vi "Test CycloneDX BOM.vi"() -> ()   [LabVIEW 2017]
uses:
  CycloneDX/CycloneDX JSON/CycloneDX Types.ctl
  <vilib>/National Instruments/NIPM API (Beta)/_support/package attributes.ctl
  <vilib>/JKI/VIPM API/command-line/support/Library Contents Cluster_vipm_api.ctl
  CycloneDX/CycloneDX SBOM/CycloneDX SBOM.lvclass
  C:/LabVIEW Working Directory/labview-cyclonedx-sbom/Source/CycloneDX/CycloneDX JSON/CycloneDX JSON.lvclass
  CycloneDX/CycloneDX Component/CycloneDX Component.lvclass
  CycloneDX/CycloneDX JSON/CycloneDX JSON.lvclass
  <vilib>/JKI/VIPM API/VIPM API_vipm_api.lvlib
  <vilib>/National Instruments/NIPM API (Beta)/NIPM_API.lvlib
  VIP Support/VIP SBOM Support.lvlib
  NIPKG Support/NIPKG SBOM Support.lvlib
  <vilib>/JDP Science/JSONtext/JSONtext.lvlib
panel:
  out "error out":errorcluster
  out "JSON":string="{\r  \"bomFormat\":\"CycloneDX\",\r  \"specVersion\":\"1.5\",\r  \"serialNumber\":\"urn:uuid:dd314ffc-d076-4662-b32e-20b770deedce\",\r  \"metadata\":{\r    \"timestamp\":\"2024-08-06T15:38:24.581Z\",\r    \"manufacture\":{\"name\":\"MySoftwareCompany Ltd\"},\r    \"supplier\":{\"name\":\"MySoftwareCompany Ltd\"},\r    \"component\":{\r      \"type\":\"application\",\r      \"name\":\"softwarename\",\r      \"metadata\":{\r        \"component\":{\r          \"supplier\":{\"name\":\"MySoftwareCompany Ltd\"},\r          \"author\":{\"name\":\"MySoftwareCompany Ltd\"},\r          \"version\":\"1.0.0\",\r          \"description\":\"My Software Name - the best software available\",\r          \"cpe\":\"cpe:2.3:a:mysoftwarecompany:softwarename:1.2.219:*:*:*:*:*:*:*\"\r        }\r      }\r    }\r  },\r  \"components\":[\r    {\r      \"type\":\"library\",\r      \"name\":\"MGI Numeric\",\r      \"version\":\"1.1.0.2\",\r      \"publisher\":\"MGI\",\r      \"author\":\"MGI\",\r      \"purl\":\"pkg:vip/MGI/mgi_lib_numeric@1.1.0.2?repository_name=NI%20LabVIEW%20Tools%20Network\",\r      \"licenses\":[\r        {\r          \"id\":\"BSD-3-Clause\",\r          \"name\":\"BSD 3-Clause \\\"New\\\" or \\\"Revised\\\" License\"\r        }\r      ],\r      \"properties\":[\r        {\r          \"name\":\"packageName\",\r          \"value\":\"mgi_lib_numeric-1.1.0.2\"\r        },\r        {\r          \"name\":\"repositoryName\",\r          \"value\":\"NI LabVIEW Tools Network\"\r        }\r      ]\r    },\r    {\r      \"type\":\"platform\",\r      \"name\":\"ni-labview-2021-runtime-engine-x86\",\r      \"version\":\"21.1.0.49476-0+f324\",\r      \"author\":\"National Instruments\",\r      \"description\":\"The LabVIEW Runtime is a software add-on that enables engineers to run executables on a nondevelopment machine.\",\r      \"purl\":\"pkg:nipkg/National%20Instruments/ni-labview-2021-runtime-engine-x86@21.1.0.49476-0+f324\",\r      \"properties\":[\r        {\r          \"name\":\"maintainerEmail\",\r          \"value\":\"support@ni.com\"\r        },\r        {\r          \"name\":\"homepage\",\r          \"value\":\"https://www.ni.com\"\r        },\r        {\r          \"name\":\"displayVersion\",\r          \"value\":\"2021 SP1\"\r        },\r        {\r          \"name\":\"displayName\",\r          \"value\":\"LabVIEW Runtime (32-bit)\"\r        },\r        {\r          \"name\":\"architecture\",\r          \"value\":\"windows_x64\"\r        },\r        {\r          \"name\":\"packageSizeBytes\",\r          \"value\":\"29378434\"\r        },\r        {\r          \"name\":\"detailedDescription\",\r          \"value\":\"The LabVIEW Runtime enables you to run executables created with the LabVIEW Application Builder on machines that do not have LabVIEW installed. The LabVIEW Runtime includes the libraries and other files necessary to run basic application types built in LabVIEW.\"\r        }\r      ]\r    }\r  ]\r}"
  # "Example CycloneDX SBOM Generation using constant(s) for dependencies"
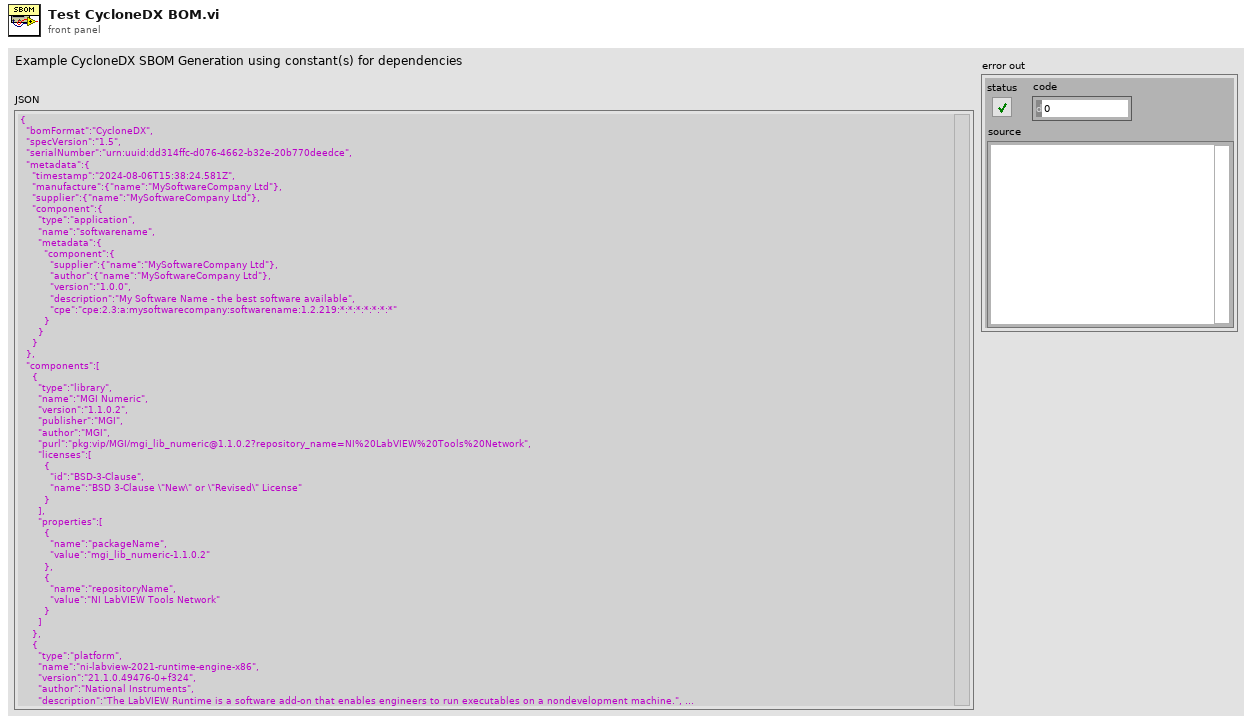
[diagram p1: front panel]
types:
  T1 = typedef "VIPM API_vipm_api.lvlib/Library Contents Cluster_vipm_api.ctl" = cluster{"Package Name":string, "Version":string, "Display Name":string, "Repository Name":string, "Company Name":string, "License Type":string, "Installed":bool, "Deprecated":bool, "Dependency or Conflict Problem":bool, "Downloaded":bool}
  T2 = typedef "NIPM_API.lvlib/package attributes.ctl" = cluster{"Package Name":string, "Display name":string, "Version":string, "Display version":string, "Synopsis":string, "Description":string, "Maintainer":string, "Maintainer email address":string, "Category":string, "Homepage":string, "Release notes":string, "Depends":string[], "Recommends":string[], "Suggests":string[], "Conflicts":string[], "Provides":string[], "Replaces":string[], "Supplements":string[], "Enhances":string[], "Product":bool, "User visible":bool, "Installed size (KB)":u64, "Package filesize (bytes)":u64, "Architecture":string, "Agent":string, "MD5Checksum":string}
  T3 = typedef "LabVIEW CycloneDX SBOM.lvlib/CycloneDX JSON.lvclass/CycloneDX Types.ctl" = enum16{"application", "framework", "library", "container", "platform", "operating-system", "device", "device-driver", "firmware", "file", "machine-learning-model", "data"}
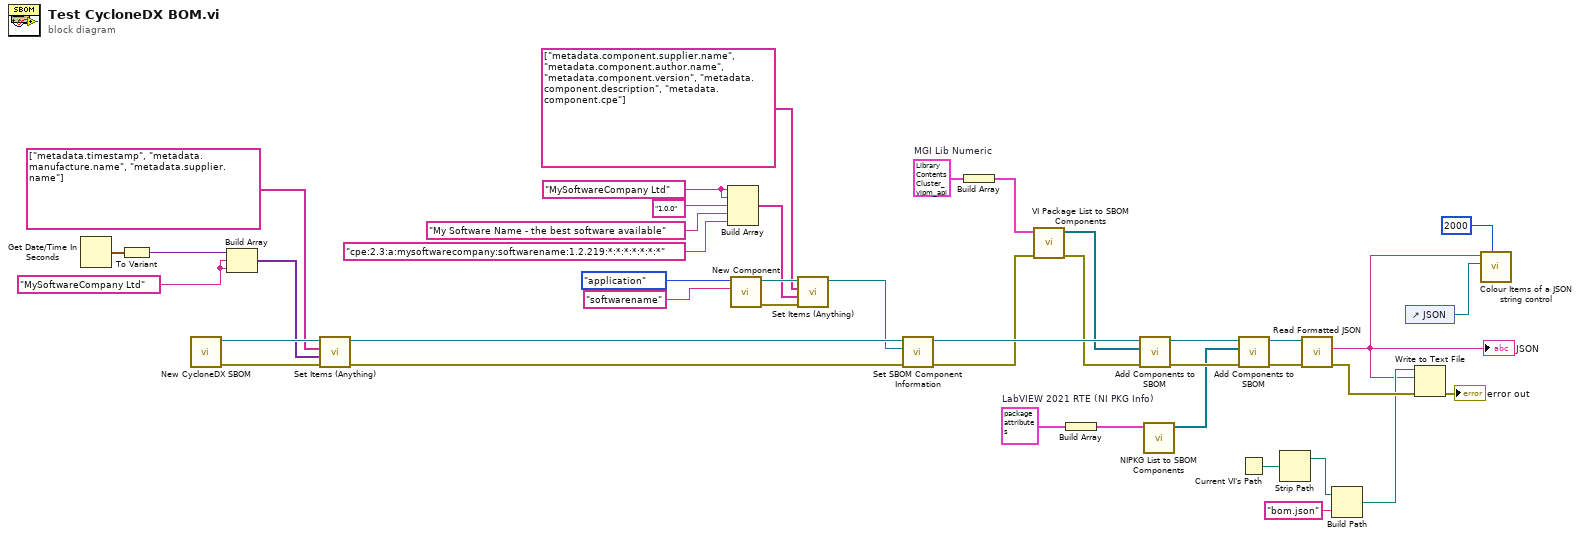
[diagram p0: block diagram]
diagram:
  w2 = T1 {"Package Name"="mgi_lib_numeric-1.1.0.2", "Version"="1.1.0.2", "Display Name"="MGI Numeric", "Repository Name"="NI LabVIEW Tools Network", "Company Name"="MGI", "License Type"="BSD", "Installed"=TRUE, "Deprecated"=FALSE, "Dependency or Conflict Problem"=FALSE, "Downloaded"=TRUE}  # MGI Lib Numeric
  w4 = T2 {"Package Name"="ni-labview-2021-runtime-engine-x86", "Display name"="LabVIEW Runtime (32-bit)", "Version"="21.1.0.49476-0+f324", "Display version"="2021 SP1", "Synopsis"="The LabVIEW Runtime is a software add-on that enables engineers to run executables on a nondevelopment machine.", "Description"="The LabVIEW Runtime enables you to run executables created with the LabVIEW Application Builder on machines that do not have LabVIEW installed. The LabVIEW Runtime includes the libraries and other files necessary to run basic application types built in LabVIEW.", "Maintainer"="National Instruments", "Maintainer email address"="support@ni.com", "Category"="Programming Environments", "Homepage"="https://www.ni.com", "Release notes"="Refer to the NI website at https://www.ni.com/r/lv2021x1rm for installation instructions, known issues, bug fixes, compatibility information, and other important notices about this product.", "Depends"=["ni-activex-container (>= 17.1.2)", "ni-curl (>= 21.3.0)", "ni-deployment-framework-x86 (>= 21.0.0)", "ni-error-report-x86 (>= 20.1.0)", "ni-error-reporting-interface (>= 20.1.0)", "ni-labview-2021-realtime-nbfifo-x86 (>= 21.0.0)", "ni-labview-2021-runtime-engine-resource (>= 21.1.0)", "ni-logos (>= 21.0.0)", "ni-lv-web-server-labview-2021-runtime-engine-x86-support (>= 21.5.0)", "ni-matlab-interface (>= 21.1.0)", "ni-mdfsupport (>= 21.5.0)", "ni-mdnsresponder (>= 21.5.0)", "ni-metauninstaller (>= 21.5.0)", "ni-mkl-2017 (>= 17.0.1)", "ni-mkl-2020 (>= 20.0.0)", "ni-msiproperties (>= 21.5.0)", "ni-mstudio-cw3dgraph (>= 8.7.5)", "ni-msvcrt-2015 (>= 14.1.5)", "ni-python-interface (>= 21.1.0)", "ni-svcloc (>= 21.0.0)", "ni-systemlogging-utils (>= 20.0.0)", "ni-tdms (>= 21.1.0)", "ni-traceengine (>= 20.0.0)"], "Recommends"=[], "Suggests"=[], "Conflicts"=[], "Provides"=["0f5c3d28-ccea-37fa-af9e-554c677a3f03 (= 21.10.49476)", "251e8668-4013-3671-857c-61d46b2ac827 (= 21.10.49476)", "ni-labview-runtime-engine-x86 (= 21.1.0)", "ni-labview-2021-runtime-engine-x86 (= 21.1.0.49476-0+f324)"], "Replaces"=[], "Supplements"=[], "Enhances"=[], "Product"=TRUE, "User visible"=TRUE, "Installed size (KB)"=0, "Package filesize (bytes)"=29378434, "Architecture"="windows_x64", "Agent"="wininst", "MD5Checksum"=""}  # LabVIEW 2021 RTE (NI PKG Info)
  w22 = "MySoftwareCompany Ltd"
  w31 = "MySoftwareCompany Ltd"
  n1 = Get Date/Time In Seconds() -> (seconds since 1Jan1904=w34:timestamp)
  n2 = To Variant(anything=w34) -> (Variant=w33:variant)
  n3 = call "New CycloneDX SBOM.vi"() -> ("error out"=w37:errorcluster, "CycloneDX SBOM out"=w36:refnum<class "CycloneDX SBOM.lvclass">)  [unwired: 10 in]
  n4 = Build Array(w33, w31, w31) -> (w32:variant[])
  n5 = call "Set Items (Anything).vi"("error in (no error)"=w37, "Value"=w32, "Item Paths"=string[] ["metadata.timestamp", "metadata.manufacture.name", "metadata.supplier.name"] ("Object (or Item) Path"), "CycloneDX SBOM in"=w36) -> ("error out"=w28:errorcluster, "CycloneDX SBOM out"=w29:refnum<class "CycloneDX SBOM.lvclass">)  [unwired: 6 in]
  n6 = Build Array(w22, w22, "1.0.0", "My Software Name - the best software available", "cpe:2.3:a:mysoftwarecompany:softwarename:1.2.219:*:*:*:*:*:*:*") -> (w18:string[])
  n7 = call "New Component.vi"("name"="softwarename", "type"=CycloneDX_Types."application") -> ("error out"=w25:errorcluster, "CycloneDX Component out"=w24:refnum<class "CycloneDX Component.lvclass">)  [unwired: 8 in]
  n8 = call "Set Items (Anything).vi"("error in (no error)"=w25, "Value"=w18, "Item Paths"=string[] ["metadata.component.supplier.name", "metadata.component.author.name", "metadata.component.version", "metadata.component.description", "metadata.component.cpe"] ("Object (or Item) Path"), "CycloneDX SBOM in"=w24) -> ("CycloneDX SBOM out"=w17:refnum<class "CycloneDX Component.lvclass">)  [unwired: 6 in, 1 out]
  n9 = call "Set SBOM Component Information.vi"("error in (no error)"=w28, "CycloneDX Component"=w17, "CycloneDX SBOM in"=w29) -> ("error out"=w14:errorcluster, "CycloneDX SBOM out"=w16:refnum<class "CycloneDX SBOM.lvclass">)  [unwired: 7 in]
  n10 = Build Array(w2) -> (w1:T1[])
  n11 = call "VI Package List to SBOM Components.vi"("error in (no error)"=w14, "VIP List in"=w1) -> ("error out"=w13:errorcluster, "SBOM Components out"=w15:refnum<class "CycloneDX Component.lvclass">[])  [unwired: 8 in]
  n12 = Build Array(w4) -> (w3:T2[])
  n13 = call "Add Components to SBOM.vi"("error in (no error)"=w13, "Component(s) to add"=w15, "CycloneDX SBOM in"=w16) -> ("error out"=w11:errorcluster, "CycloneDX SBOM out"=w12:refnum<class "CycloneDX SBOM.lvclass">)  [unwired: 7 in]
  n14 = call "NIPKG List to SBOM Components.vi"("nipkg packages"=w3) -> ("SBOM Components out"=w8:refnum<class "CycloneDX Component.lvclass">[])  [unwired: 9 in, 1 out]
  n15 = call "Add Components to SBOM.vi"("error in (no error)"=w11, "Component(s) to add"=w8, "CycloneDX SBOM in"=w12) -> ("error out"=w10:errorcluster, "CycloneDX SBOM out"=w9:refnum<class "CycloneDX SBOM.lvclass">)  [unwired: 7 in]
  n16 = Current VI's Path() -> (path=w41:path)
  n17 = Strip Path(path=w41) -> (stripped path=w40:path)  [unwired: 1 out]
  n18 = call "Read Formatted JSON.vi"("error in (no error)"=w10, "CycloneDX SBOM in"=w9) -> ("error out"=w42:errorcluster, "JSON"=w5:string)  [unwired: 7 in, 1 out]
  "JSON" <- w5
  n19 = Build Path(base path=w40, name or relative path="bom.json") -> (appended path=w38:path)
  n20 = control-ref of="JSON"() -> (w6:refnum<vi>)
  n21 = Write to Text File(file (use dialog)=w38, text=w5, error in=w42) -> (error out=→"error out":errorcluster)  [unwired: 1 in, 2 out]
  n22 = call <vilib>:"Colour Items of a JSON string control.vi"("Maximum UI Property calls"=2000, "String Control"=w6, "JSON"=w5) -> ()  [unwired: 9 in]
